vi "LV86_Smooth.vi"(3 "Image in":T1 {"Dialogs" format="%.0b"}) -> (1 "Image out":T1 {"Dialogs" format="%.0b"})   [LabVIEW 2024]
doc: "This VI smooths the incoming image."
uses:
  <userlib>/ImageProcessing/QTLIB_2595_LV86/QT_Image.ctl
panel:
  # "This VI smooths the incoming image."
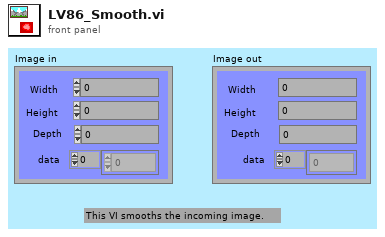
[diagram p1: front panel]
types:
  T1 = typedef "QT_Image.ctl" = cluster{"Width":i32, "Height":i32, "Depth":i32, "data":u8[], "Compressed data":u8[], "Color table":u32[], "Duration":i32, "Options":i32, "Timestamp":i32, "ID":i32, "Reserved":i32, "Dialogs":u32}
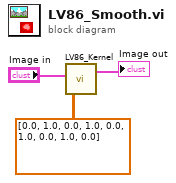
[diagram p0: block diagram]
diagram:
  n1 = call <userlib>:"LV86_Kernel.vi"("Kernel"=sgl[][] [[0.0, 1.0, 0.0], [1.0, 0.0, 1.0], [0.0, 1.0, 0.0]], "Image in"="Image in") -> ("Image out"=→"Image out":T1)  [unwired: 1 out]
